vi "_rsscope Default Instrument Setup.vi"(8 "error in (no error)":errorcluster, 11 "VISA resource name":refnum<visa-resource-name>) -> (0 "error out":errorcluster, 3 "VISA resource name out":refnum<visa-resource-name>)   [LabVIEW 2018]
doc: "This Utility VI sends a default command string to the instrument whenever a new VISA session is opened, or the instrument is reset.\nThis VI is intended to be used as a subVI for the Initialize.vi and Reset VI. Altering this VI could cause these two VI's to operate incorrectly."
uses:
  rsidr_core.llb/type_Options_Item_Parsing.ctl
  rsidr_core.llb/rsscope_rsidr_core.lvlib
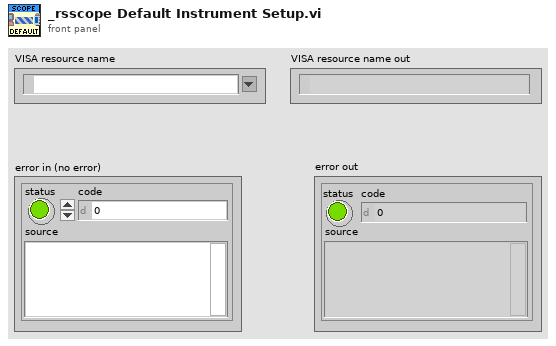
[diagram p1: front panel]
types:
  T1 = typedef "rsscope_rsidr_core.lvlib/type_Options_Item_Parsing.ctl" = enum16{"None", "Keep parts after dash", "Keep parts before dash", "Automatic"}
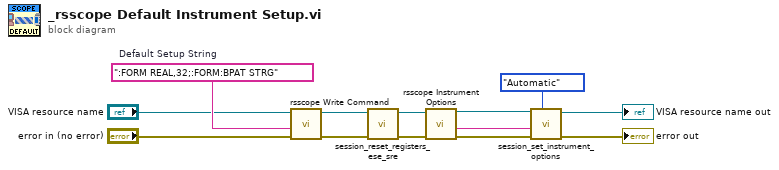
[diagram p0: block diagram]
diagram:
  w13 = ":FORM REAL,32;:FORM:BPAT STRG"  # Default Setup String
  n1 = call "rsscope Write Command.vi"("error in (no error)"="error in (no error)", "Command"=w13, "VISA resource name"="VISA resource name") -> ("error out"=w8:errorcluster, "VISA resource name out"=w7:refnum<visa-resource-name>)  [unwired: 7 in]
  n2 = call "session_reset_registers_ese_sre.vi"("error in"=w8, "VISA resource name"=w7) -> ("error out"=w6:errorcluster, "VISA resource name out"=w5:refnum<visa-resource-name>)  [unwired: 8 in]
  n3 = call "rsscope Instrument Options.vi"("VISA resource name"=w5, "error in (no error)"=w6) -> ("VISA resource name out"=w9:refnum<visa-resource-name>, "Options List"=w4:string, "error out"=w10:errorcluster)  [unwired: 9 in, 2 out]
  n4 = call "session_set_instrument_options.vi"("Item Parsing"=type_Options_Item_Parsing."Automatic", "error in"=w10, "Options string"=w4, "VISA resource name"=w9) -> ("error out"=→"error out":errorcluster, "VISA resource name out"=→"VISA resource name out":refnum<visa-resource-name>)  [unwired: 4 in, 2 out]
